vi "Append.vi"(6 "deadline":T1={"mode"=enum."Relative", "deadline (ms)"=30000}, 8 "error in (no error)":errorcluster, 10 "data":u8[](array[numeric]), 11 "Buffer Download Controller in":refnum<class "Buffer Download Controller.lvclass">) -> (0 "error out":errorcluster, 3 "Buffer Download Controller out":refnum<class "Buffer Download Controller.lvclass">)   [LabVIEW 2020, in "NI_SFTP.lvlib" / "Buffer Download Controller.lvclass"]
uses:
  <vilib>/net/SFTP/API/Support/Download/Buffer/Buffer Download Controller.lvclass
  <vilib>/Utility/Deadline/Deadline.ctl
  <vilib>/Utility/Deadline/Mode.ctl
  <vilib>/net/SFTP/API/Support/Download/Buffer/Buffer Download Controller.lvclass/Buffer Download Controller.ctl
  <vilib>/Utility/Deadline/NI_Deadline.lvlib
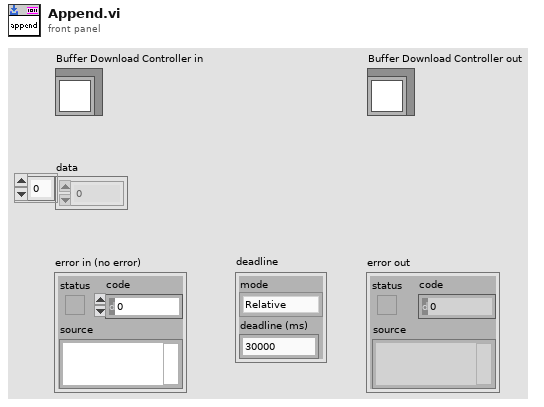
[diagram p1: front panel]
types:
  T1 = typedef "NI_Deadline.lvlib/Deadline.ctl" = cluster{"mode":T2, "deadline (ms)":u32}
  T2 = typedef "NI_Deadline.lvlib/Mode.ctl" = enum16{"Relative", "Use deadline", "Wait forever", "Nonblocking", "N/A"}
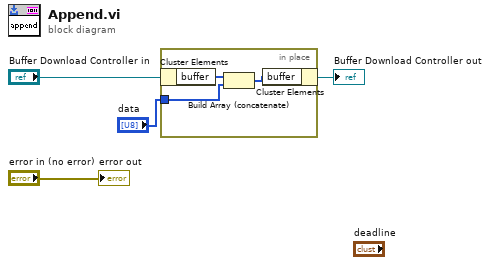
[diagram p0: block diagram]
diagram:
  n1 = in-place "In Place Element Structure" {
    in-place-border: "data" -> [w6]
    n2 = in-place-cluster #1("Buffer Download Controller in") -> ("buffer"=w7:u8[])
    n3 = Build Array (concatenate)(w7, w6) -> (w5:u8[])
    n4 = in-place-cluster #1("buffer"=w5) -> (→"Buffer Download Controller out":refnum<class "Buffer Download Controller.lvclass">)
  }
  "error out" <- "error in (no error)"
